vi "TIO RPC Notification.vi"(4 "Notification Prefix":string, 5 "Timeout in ms":i32=1000, 7 "error in (no error)":errorcluster, 9 "Payload":string, 10 "Topic":string) -> (0 "error out":errorcluster, 2 "REP":string, 3 "Response":bool)   [LabVIEW 2016]
panel:
  out "timed out?":bool
  out "Topic 2":string
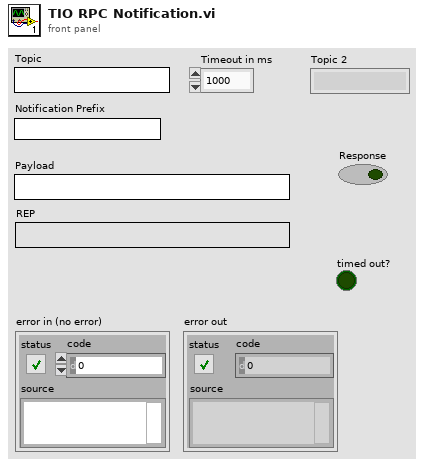
[diagram p1: front panel]
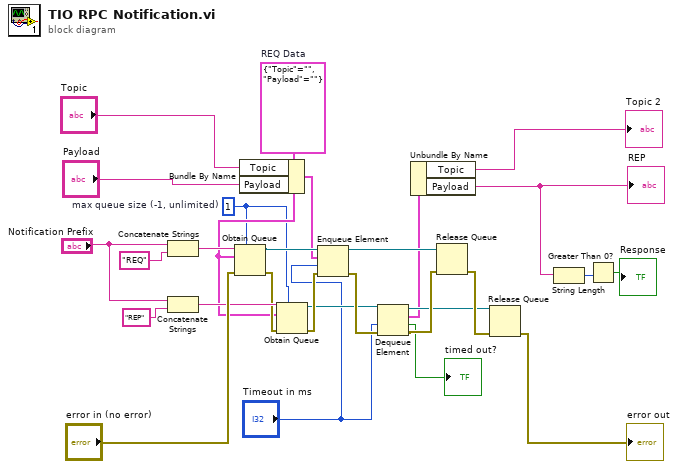
[diagram p0: block diagram]
diagram:
  w1 = 1  # max queue size (-1, unlimited)
  w15 = cluster{"Topic":string, "Payload":string} {"Topic"="", "Payload"=""}  # REQ Data
  n1 = Concatenate Strings("Notification Prefix", "REQ" ("name (unnamed)")) -> (w19:string)
  n2 = Concatenate Strings("Notification Prefix", "REP" ("name (unnamed)")) -> (w17:string)
  n3 = Obtain Queue(max queue size (-1, unlimited)=w1, name (unnamed)=w19, element data type=w15, error in (no error)="error in (no error)") -> (queue out=w14:refnum<queue>, error out=w16:errorcluster)  [unwired: 1 in, 1 out]
  n4 = Bundle By Name(cluster=w15, "Topic"="Topic", "Payload"="Payload") -> (w3:cluster{"Topic":string, "Payload":string})
  n5 = Obtain Queue(max queue size (-1, unlimited)=w1, name (unnamed)=w17, element data type=w15, error in (no error)=w16) -> (queue out=w9:refnum<queue>, error out=w13:errorcluster)  [unwired: 1 in, 1 out]
  n6 = Enqueue Element(queue=w14, element=w3, timeout in ms (-1)="Timeout in ms", error in (no error)=w13) -> (queue out=w7:refnum<queue>, error out=w12:errorcluster)  [unwired: 1 out]
  n7 = Dequeue Element(queue=w9, timeout in ms (-1)="Timeout in ms", error in (no error)=w12) -> (queue out=w8:refnum<queue>, element=w5:cluster{"Topic":string, "Payload":string}, timed out?=→"timed out?":bool, error out=w11:errorcluster)
  n8 = Unbundle By Name(w5) -> ("Topic"=→"Topic 2":string, "Payload"=w25:string)
  "REP" <- w25
  n9 = Release Queue(queue=w7, error in (no error)=w11) -> (error out=w10:errorcluster)  [unwired: 1 in, 2 out]
  n10 = Release Queue(queue=w8, error in (no error)=w10) -> (error out=→"error out":errorcluster)  [unwired: 1 in, 2 out]
  n11 = String Length(string=w25) -> (length=w24:i32)
  n12 = Greater Than 0?(x=w24) -> (x > 0?=→"Response":bool)
